vi "Copy Data.vi"(7 "num_frames":u64, 8 "error in (no error)":errorcluster, 9 "sample_rate":u32, 10 "channels":u32, 11 "Data Pointer in":i64) -> (0 "error out":errorcluster, 2 "Waveform Data":waveform(i16)[](array[waveform]), 3 "Data Pointer out":i64)   [LabVIEW 2020, in "G-Audio.lvlib"]
doc: "Copies the audio data allocated by a DLL into LabVIEW. Assumes data is interleaved I16 format."
uses:
  G-Audio.lvlib
  9030b790-3ef4-4341-af47-ee342ff8418a.vi
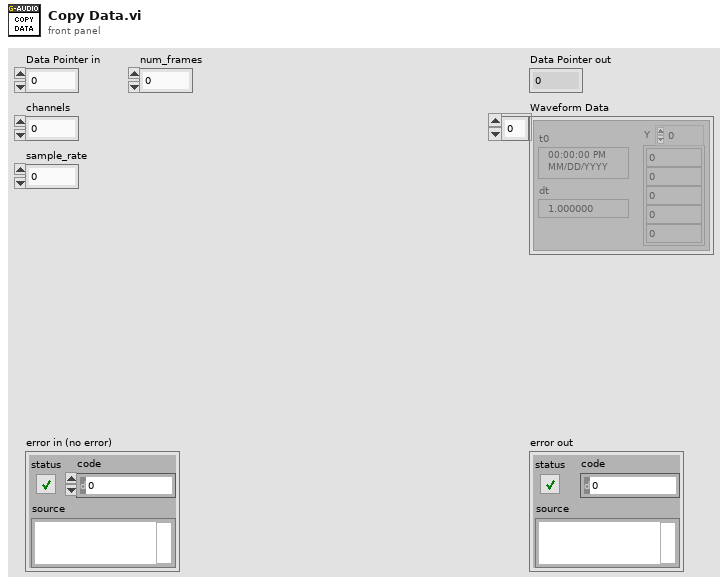
[diagram p1: front panel]
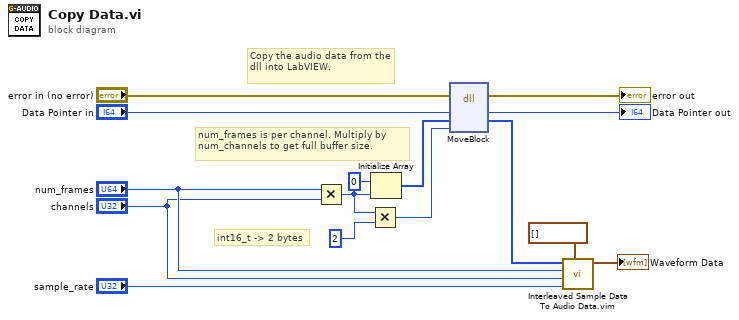
[diagram p0: block diagram]
diagram:
  # "num_frames is per channel. Multiply by num_channels to get full buffer size."
  # "Copy the audio data from the dll into LabVIEW."
  # "int16_t -> 2 bytes"
  n1 = Multiply(x="num_frames", y="channels") -> (x*y=w9:u64)
  n2 = Multiply(x=w9, y=u64 2) -> (x*y=w12:u64)
  n3 = Initialize Array(i16 0 ("num_samples"), w9) -> (w14:i16[])
  n4 = dll-call lib="LabVIEW" fn="MoveBlock"(error in="error in (no error)", "Address (Pointer)"="Data Pointer in", "Destination"=w14, "Size"=w12) -> (error out=→"error out":errorcluster, "Address (Pointer)"=→"Data Pointer out":i64, "Destination"=w6:i16[])  [unwired: 4 in, 1 out]
  n5 = call "Interleaved Sample Data To Audio Data.vim"("Data Format"=waveform(i16)[] [], "sample_rate"="sample_rate", "channels"="channels", "num_frames"="num_frames", "sample_data"=w6) -> ("Audio Data"=→"Waveform Data":waveform(i16)[])  [unwired: 6 in]
